vi "快捷菜单激活(波形图表).vi"(11 "菜单引用":refnum<k9>) -> ()   [LabVIEW 2021]
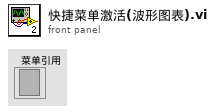
[diagram p1: front panel]
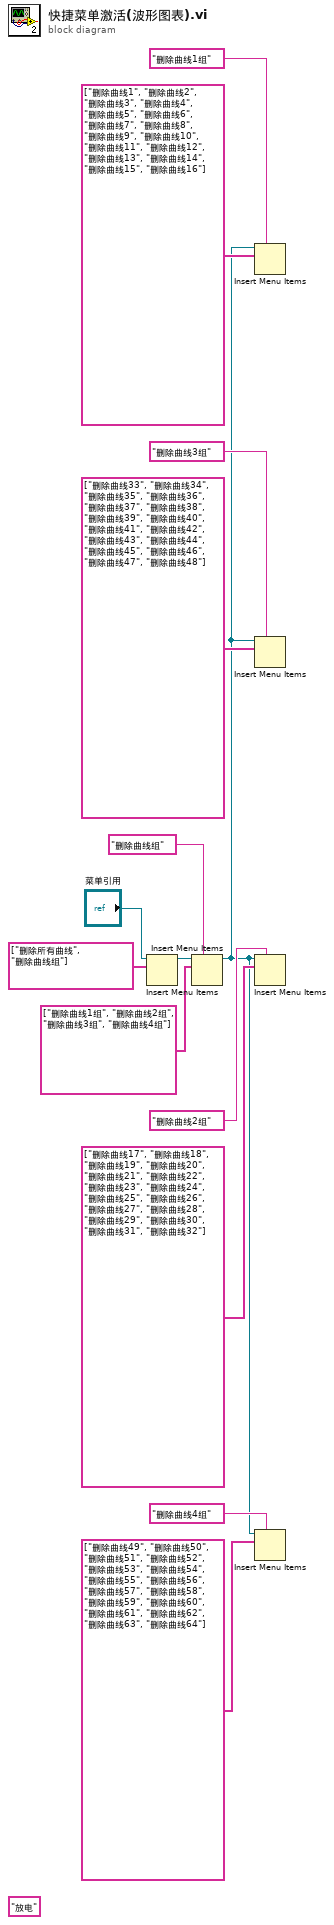
[diagram p0: block diagram]
diagram:
  (unwired) "放电" ("菜单标识符")
  n1 = Insert Menu Items ("插入菜单项")(8:string[] ["删除所有曲线", "删除曲线组"] ("项名称"), 9:"菜单引用") -> (3:w11:refnum<k9>)  [unwired: 4 in, 2 out]
  n2 = Insert Menu Items ("插入菜单项")(5:"删除曲线组" ("菜单标识符"), 8:string[] ["删除曲线1组", "删除曲线2组", "删除曲线3组", "删除曲线4组"] ("项名称"), 9:w11) -> (3:w1:refnum<k9>)  [unwired: 3 in, 2 out]
  n3 = Insert Menu Items ("插入菜单项")(5:"删除曲线1组" ("菜单标识符"), 8:string[] ["删除曲线1", "删除曲线2", "删除曲线3", "删除曲线4", "删除曲线5", "删除曲线6", "删除曲线7", "删除曲线8", "删除曲线9", "删除曲线10", "删除曲线11", "删除曲线12", "删除曲线13", "删除曲线14", "删除曲线15", "删除曲线16"] ("项名称"), 9:w1) -> ()  [unwired: 3 in, 3 out]
  n4 = Insert Menu Items ("插入菜单项")(5:"删除曲线3组" ("菜单标识符"), 8:string[] ["删除曲线33", "删除曲线34", "删除曲线35", "删除曲线36", "删除曲线37", "删除曲线38", "删除曲线39", "删除曲线40", "删除曲线41", "删除曲线42", "删除曲线43", "删除曲线44", "删除曲线45", "删除曲线46", "删除曲线47", "删除曲线48"] ("项名称"), 9:w1) -> ()  [unwired: 3 in, 3 out]
  n5 = Insert Menu Items ("插入菜单项")(5:"删除曲线2组" ("菜单标识符"), 8:string[] ["删除曲线17", "删除曲线18", "删除曲线19", "删除曲线20", "删除曲线21", "删除曲线22", "删除曲线23", "删除曲线24", "删除曲线25", "删除曲线26", "删除曲线27", "删除曲线28", "删除曲线29", "删除曲线30", "删除曲线31", "删除曲线32"] ("项名称"), 9:w1) -> ()  [unwired: 3 in, 3 out]
  n6 = Insert Menu Items ("插入菜单项")(5:"删除曲线4组" ("菜单标识符"), 8:string[] ["删除曲线49", "删除曲线50", "删除曲线51", "删除曲线52", "删除曲线53", "删除曲线54", "删除曲线55", "删除曲线56", "删除曲线57", "删除曲线58", "删除曲线59", "删除曲线60", "删除曲线61", "删除曲线62", "删除曲线63", "删除曲线64"] ("项名称"), 9:w1) -> ()  [unwired: 3 in, 3 out]
